vi "sort channels.vi"(8 "error in":errorcluster, 11 "channels in":refnum<class "TBM channel.lvclass">[](array[class])) -> (0 "error out":errorcluster, 2 "data allocations":T1, 3 "channels out":refnum<class "TBM channel.lvclass">[](array[class]))   [LabVIEW 2013, in "TBM channel.lvclass"]
doc: "Sorts all channels by classification and allocates a data interface for each."
uses:
  TBM channel.lvclass
  data tables.ctl
  <vilib>/NI/Tag Bus/dictionary/data dictionary.lvclass
  <vilib>/NI/Tag Bus/dictionary table pair.ctl
  <vilib>/NI/Tag Bus/table/data table.ctl
  <vilib>/NI/Tag Bus/tag/tag descriptor.lvclass
  TBM channel.lvclass/TBM channel.ctl
  <vilib>/NI/Tag Bus/dictionary/data dictionary.lvclass/data dictionary.ctl
  <vilib>/NI/Tag Bus/tag bus.lvlib
  <vilib>/NI/Tag Bus/table/data table.lvlib
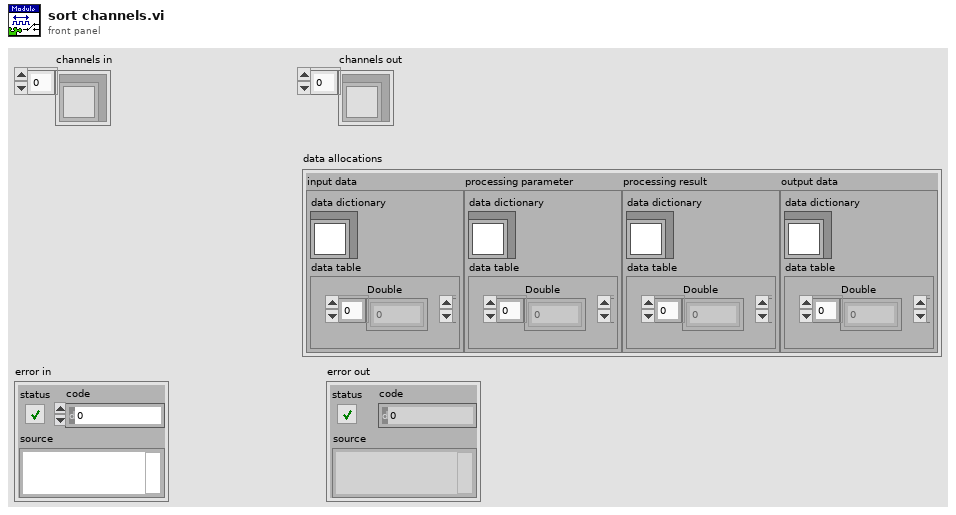
[diagram p1: front panel]
types:
  T1 = typedef "TBM channel.lvclass/data tables.ctl" = cluster{"input data":T2, "processing parameter":T2, "processing result":T2, "output data":T2}
  T2 = typedef "tag bus.lvlib/dictionary table pair.ctl" = cluster{"data dictionary":refnum<class "data dictionary.lvclass">, "data table":T3}
  T3 = typedef "tag bus.lvlib/data table.lvlib/data table.ctl" = cluster{"Double":dbl[], "Single":sgl[], "I64":i64[], "I32":i32[], "I16":i16[], "I8":i8[], "U64":u64[], "U32":u32[], "U16":u16[], "U8":u8[], "Boolean":bool[], "String":string[], "Array of Double":cluster{"DBL Array":dbl[]}[], "Array of Single":cluster{"SGL Array":sgl[]}[], "Array of I64":cluster{"I64 Array":i64[]}[], "Array of I32":cluster{"I32 Array":i32[]}[], "Array of I16":cluster{"I16 Array":i16[]}[], "Array of I8":cluster{"I8 Array":i8[]}[], "Array of U64":cluster{"U64 Array":u64[]}[], "Array of U32":cluster{"U32 Array":u32[]}[], "Array of U16":cluster{"U16 Array":u16[]}[], "Array of U8":cluster{"U8 Array":u8[]}[], "Array of Boolean":cluster{"Boolean Array":bool[]}[], "Array of String":cluster{"String Array":string[]}[]}
  T4 = typedef "TBM channel.lvclass/channel classification.ctl" = enum16{"input data", "output data", "processing parameter", "processing result"}
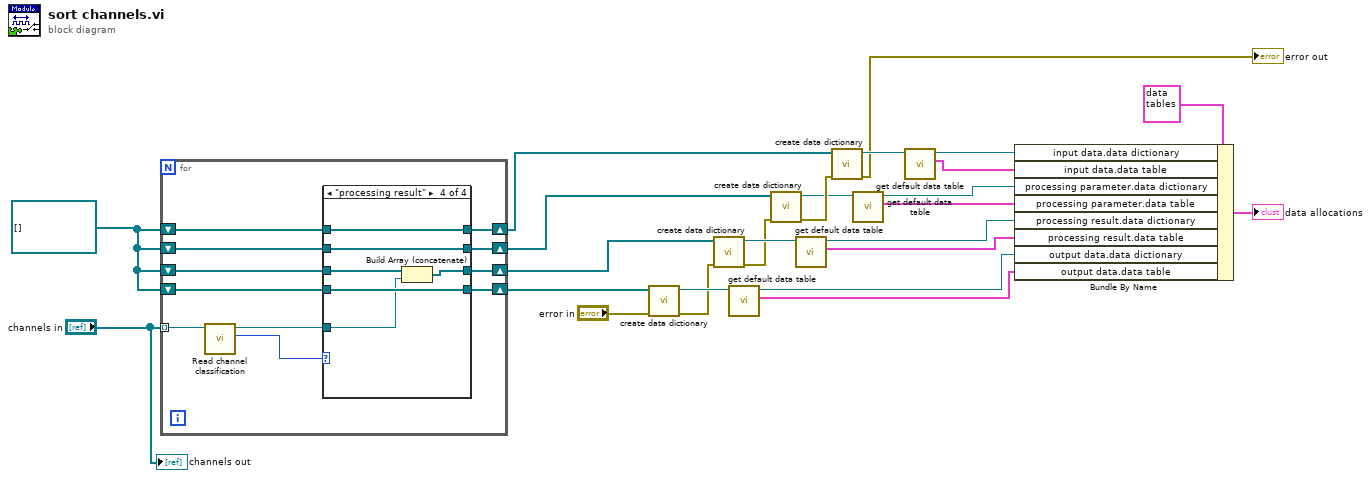
[diagram p0: block diagram]
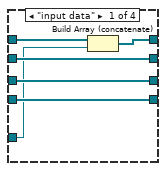
[diagram p2: hidden frame]
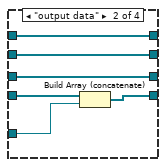
[diagram p3: hidden frame]
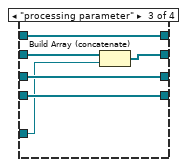
[diagram p4: hidden frame]
diagram:
  w14 = refnum<class "tag descriptor.lvclass">[] []
  n1 = for {
    tunnel: "channels in" -> [w27] mode=indexing
    shift-right: [w36] -> w3
    shift-left: w14 -> [w35]
    shift-right: [w34] -> w2
    shift-left: w14 -> [w33]
    shift-right: [w31] -> w1
    shift-left: w14 -> [w32]
    shift-right: [w30] -> w12
    shift-left: w14 -> [w29]
    n2 = call "Read channel classification.vi"("channel in"=w27) -> ("channel classification"=w28:T4, "channel out"=w26:refnum<class "TBM channel.lvclass">)  [unwired: 8 in, 1 out]
    n3 = case shown="\"processing result\"" w28 {
      tunnel: [w38 w47 w53 w60] -> w36
      tunnel: w35 -> [w39 w47 w53 w60]
      tunnel: [w42 w46 w50 w59] -> w34
      tunnel: w33 -> [w42 w46 w51 w59]
      tunnel: w32 -> [w41 w48 w52 w57]
      tunnel: [w41 w48 w52 w56] -> w31
      tunnel: [w40 w43 w54 w58] -> w30
      tunnel: w29 -> [w40 w45 w54 w58]
      tunnel: w26 -> [w37 w44 w49 w55]
      frame "input data" {
        n4 = Build Array (concatenate)(w39, w37) -> (w38:refnum<class "tag descriptor.lvclass">[])
      }
      frame "output data" {
        n5 = Build Array (concatenate)(w45, w44) -> (w43:refnum<class "tag descriptor.lvclass">[])
      }
      frame "processing parameter" {
        n6 = Build Array (concatenate)(w51, w49) -> (w50:refnum<class "tag descriptor.lvclass">[])
      }
      frame "processing result" {
        n7 = Build Array (concatenate)(w57, w55) -> (w56:refnum<class "tag descriptor.lvclass">[])
      }
    }
  }
  n8 = call <vilib>:"create data dictionary.vi"("error in"="error in", "system tags"=w12) -> ("error out"=w5:errorcluster, "data dictionary"=w11:refnum<class "data dictionary.lvclass">)  [unwired: 8 in]
  n9 = call <vilib>:"create data dictionary.vi"("error in"=w5, "system tags"=w1) -> ("error out"=w6:errorcluster, "data dictionary"=w10:refnum<class "data dictionary.lvclass">)  [unwired: 8 in]
  n10 = call <vilib>:"get default data table.vi"("data dictionary in"=w11) -> ("default data table"=w22:T3, "data dictionary out"=w23:refnum<class "data dictionary.lvclass">)  [unwired: 9 in]
  n11 = call <vilib>:"create data dictionary.vi"("error in"=w6, "system tags"=w2) -> ("error out"=w7:errorcluster, "data dictionary"=w4:refnum<class "data dictionary.lvclass">)  [unwired: 8 in]
  n12 = call <vilib>:"get default data table.vi"("data dictionary in"=w10) -> ("default data table"=w21:T3, "data dictionary out"=w20:refnum<class "data dictionary.lvclass">)  [unwired: 9 in]
  n13 = call <vilib>:"create data dictionary.vi"("error in"=w7, "system tags"=w3) -> ("error out"=→"error out":errorcluster, "data dictionary"=w9:refnum<class "data dictionary.lvclass">)  [unwired: 8 in]
  n14 = call <vilib>:"get default data table.vi"("data dictionary in"=w4) -> ("default data table"=w19:T3, "data dictionary out"=w18:refnum<class "data dictionary.lvclass">)  [unwired: 9 in]
  n15 = call <vilib>:"get default data table.vi"("data dictionary in"=w9) -> ("default data table"=w17:T3, "data dictionary out"=w16:refnum<class "data dictionary.lvclass">)  [unwired: 9 in]
  n16 = Bundle By Name(cluster=T1 {"input data"={"data dictionary"=refnum, "data table"={"Double"=[], "Single"=[], "I64"=[], "I32"=[], "I16"=[], "I8"=[], "U64"=[], "U32"=[], "U16"=[], "U8"=[], "Boolean"=[], "String"=[], "Array of Double"=[], "Array of Single"=[], "Array of I64"=[], "Array of I32"=[], "Array of I16"=[], "Array of I8"=[], "Array of U64"=[], "Array of U32"=[], "Array of U16"=[], "Array of U8"=[], "Array of Boolean"=[], "Array of String"=[]}}, "processing parameter"={"data dictionary"=refnum, "data table"={"Double"=[], "Single"=[], "I64"=[], "I32"=[], "I16"=[], "I8"=[], "U64"=[], "U32"=[], "U16"=[], "U8"=[], "Boolean"=[], "String"=[], "Array of Double"=[], "Array of Single"=[], "Array of I64"=[], "Array of I32"=[], "Array of I16"=[], "Array of I8"=[], "Array of U64"=[], "Array of U32"=[], "Array of U16"=[], "Array of U8"=[], "Array of Boolean"=[], "Array of String"=[]}}, "processing result"={"data dictionary"=refnum, "data table"={"Double"=[], "Single"=[], "I64"=[], "I32"=[], "I16"=[], "I8"=[], "U64"=[], "U32"=[], "U16"=[], "U8"=[], "Boolean"=[], "String"=[], "Array of Double"=[], "Array of Single"=[], "Array of I64"=[], "Array of I32"=[], "Array of I16"=[], "Array of I8"=[], "Array of U64"=[], "Array of U32"=[], "Array of U16"=[], "Array of U8"=[], "Array of Boolean"=[], "Array of String"=[]}}, "output data"={"data dictionary"=refnum, "data table"={"Double"=[], "Single"=[], "I64"=[], "I32"=[], "I16"=[], "I8"=[], "U64"=[], "U32"=[], "U16"=[], "U8"=[], "Boolean"=[], "String"=[], "Array of Double"=[], "Array of Single"=[], "Array of I64"=[], "Array of I32"=[], "Array of I16"=[], "Array of I8"=[], "Array of U64"=[], "Array of U32"=[], "Array of U16"=[], "Array of U8"=[], "Array of Boolean"=[], "Array of String"=[]}}} ("data allocations"), "input data.data dictionary"=w16, "input data.data table"=w17, "processing parameter.data dictionary"=w18, "processing parameter.data table"=w19, "processing result.data dictionary"=w20, "processing result.data table"=w21, "output data.data dictionary"=w23, "output data.data table"=w22) -> (→"data allocations":T1)
  "channels out" <- "channels in"
